vi "WFS Get Exposure Time Range.vi"(8 "error in (no error)":errorcluster {"code" format="%.0x"}, 11 "instrument handle":refnum<visa-resource-name>) -> (0 "error out":errorcluster {"code" format="%.0x"}, 1 "Exposure Time Max":dbl, 2 "Exposure Time Min":dbl, 3 "instrument handle out":refnum<visa-resource-name>, 4 "Exposure Time Incr":dbl)   [LabVIEW 2020]
doc: "This VI returns the available exposure range of the WFS camera in ms. The range may depend on the camera resolution set by VI ConfigureCam."
uses:
  WFS_32.dll
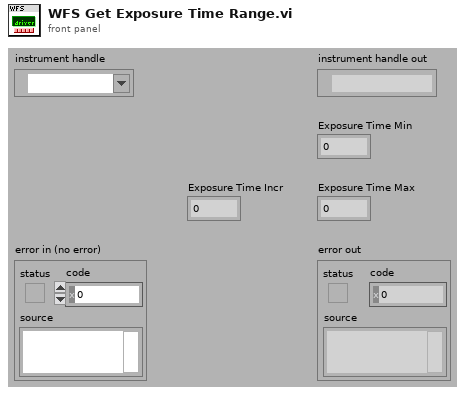
[diagram p1: front panel]
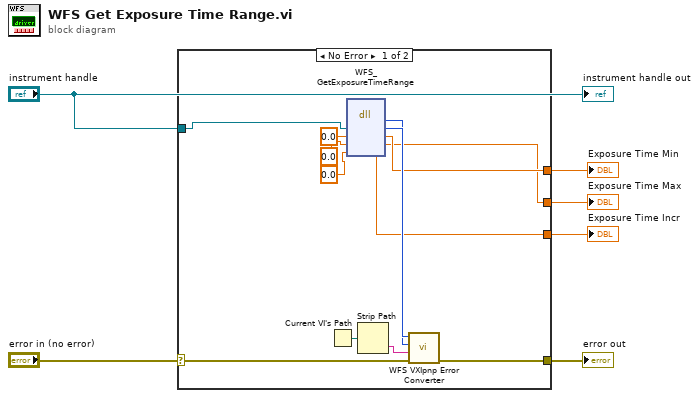
[diagram p0: block diagram]
diagram:
  n1 = case shown="No Error" "error in (no error)" {
    selector: "error in (no error)" -> [w14 w20]
    tunnel: [w13 w20] -> w6
    tunnel: "instrument handle" -> [w18 _]
    tunnel: [w11 _] -> w3
    tunnel: [w9 _] -> w2
    tunnel: [w7 _] -> w1
    frame No Error {
      n2 = Current VI's Path() -> (path=w19:path)
      n3 = dll-call lib="WFS_*.*" fn="WFS_GetExposureTimeRange"("Instrument Handle"=w18, "Exposure Time Min"=0.0, "Exposure Time Max"=0.0, "Exposure Time Incr"=0.0) -> (w16:i32, "Instrument Handle"=w17:u32, "Exposure Time Min"=w11:dbl, "Exposure Time Max"=w9:dbl, "Exposure Time Incr"=w7:dbl)  [unwired: 3 in, 2 out]
      n4 = Strip Path(path=w19) -> (name=w15:string)  [unwired: 1 out]
      n5 = call "WFS VXIpnp Error Converter.vi"("error in (no error)"=w14, "Name Of VI (\"\")"=w15, "CVI Error Code (0)"=w16, "instrument handle"=w17) -> ("error out"=w13:errorcluster)  [unwired: 6 in, 1 out]
    }
    frame Error {
    }
  }
  "error out" <- w6
  "Exposure Time Min" <- w3
  "Exposure Time Max" <- w2
  "Exposure Time Incr" <- w1
  "instrument handle out" <- "instrument handle"
